vi "Init.vi"(8 "error in (no error)":errorcluster caption="Fehler (Eingang, kein Fehler)", 11 "Data IN":T1) -> (0 "error out":errorcluster caption="Fehler (Ausgang)", 3 "Data Out":T1)   [LabVIEW 2020, in "Hardware B.lvlib"]
uses:
  Hardware B.lvlib
  Data.ctl
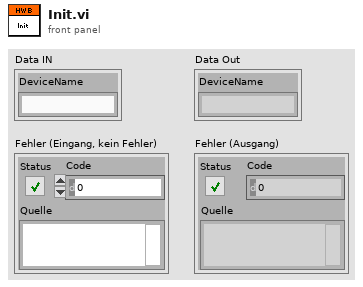
[diagram p1: front panel]
types:
  T1 = typedef "Hardware B.lvlib/Data.ctl" = cluster{"DeviceName":string}
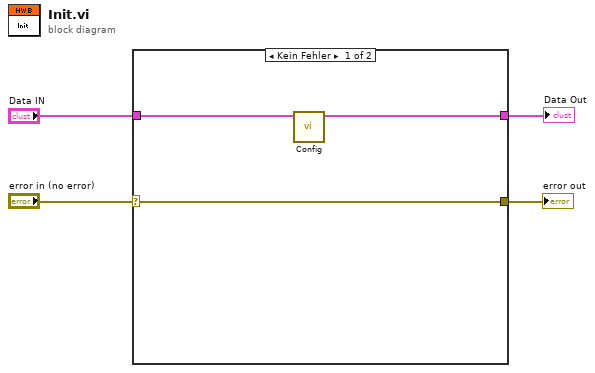
[diagram p0: block diagram]
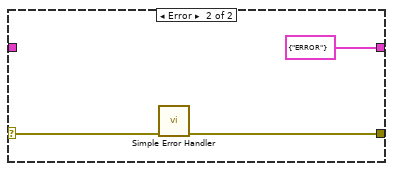
[diagram p2: hidden frame]
diagram:
  n1 = case shown="Kein Fehler" "error in (no error)" {
    selector: "error in (no error)" -> [w7 w10]
    tunnel: [w7 w9] -> w3
    tunnel: "Data IN" -> [w6 _]
    tunnel: [w5 cluster{"DeviceName":string} {"DeviceName"="ERROR"} ("Data IN")] -> w1
    frame No Error {
      n2 = call "Config.vi"("Data IN"=w6) -> ("Data Out"=w5:T1)  [unwired: 9 in, 1 out]
    }
    frame Error {
      n3 = call <vilib>:"Simple Error Handler.vi"("error in (no error)"=w10) -> ("error out"=w9:errorcluster)  [unwired: 4 in, 4 out]
    }
  }
  "error out" <- w3
  "Data Out" <- w1
